vi "Flywheel_Notifier_Begin.vi"   [LabVIEW 2020]
uses:
  Subsystems/Flywheel/Flywheel_Cluster.ctl
  Subsystems/Flywheel/Flywheel_States.ctl
  Globals/Flywheel_Globals.vi
types:
  T1 = typedef "Flywheel_Cluster.ctl" = cluster{"Flywheel_Throttle":dbl, "Control_States":T2, "Auto_Speed":bool, "Flywheel_On":bool, "Parameter_1":dbl, "Parameter_2":dbl, "Auto_Notifier":refnum<notifier>, "Step":dbl}
  T2 = typedef "Flywheel_States.ctl" = enum16{"No-Op", "Percent_Voltage", "Speed_Control_Manual", "Speed_Control_Auto", "Command_SpinUp", "Command_SpinUpAuto"}
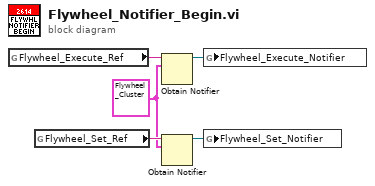
[diagram p0: block diagram]
diagram:
  w3 = T1 {"Flywheel_Throttle"=0.0, "Control_States"=enum."No-Op", "Auto_Speed"=FALSE, "Flywheel_On"=FALSE, "Parameter_1"=0.0, "Parameter_2"=0.0, "Auto_Notifier"=refnum, "Step"=0.0} ("Flywheel_Cluster")
  n1 = global read "Flywheel_Globals.vi" "Flywheel_Execute_Ref"() -> (w5:string)
  n2 = global read "Flywheel_Globals.vi" "Flywheel_Set_Ref"() -> (w4:string)
  n3 = Obtain Notifier(name (unnamed)=w5, notification data type=w3) -> (notifier out=w2:refnum<notifier>)  [unwired: 2 in, 2 out]
  n4 = Obtain Notifier(name (unnamed)=w4, notification data type=w3) -> (notifier out=w1:refnum<notifier>)  [unwired: 2 in, 2 out]
  n5 = global write "Flywheel_Globals.vi" "Flywheel_Execute_Notifier"(w2) -> ()
  n6 = global write "Flywheel_Globals.vi" "Flywheel_Set_Notifier"(w1) -> ()
